vi "To Bin.vi"(8 "error in (no error)":errorcluster, 10 "s":string, 11 "n":i32) -> (0 "error out":errorcluster, 3 "Return":i32)   [LabVIEW 2010, in "TPVG_DLL.lvlib"]
doc: "This function convert an ASCII hex of 1 to four symbols to an\ninteger\n\n\nint CLASS_DECLSPEC ToBin( int, char* );"
uses:
  TPVG_DLL.lvlib
  TPVG_DLL.dll
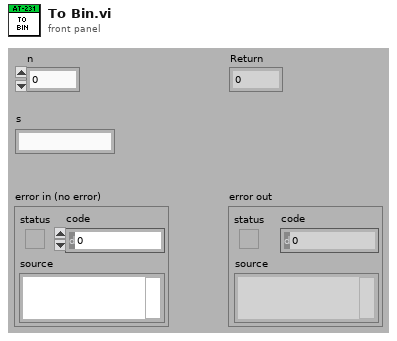
[diagram p1: front panel]
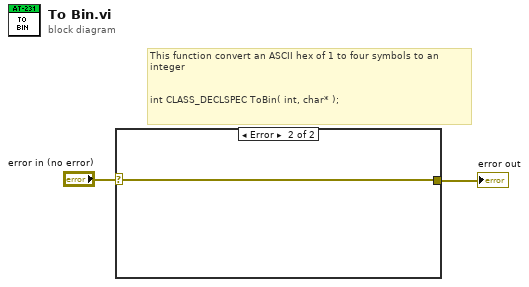
[diagram p0: block diagram]
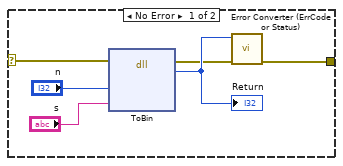
[diagram p2: hidden frame]
diagram:
  # "This function convert an ASCII hex of 1 to four symbols to an\ninteger\n\n\nint CLASS_DECLSPEC ToBin( int, char* );"
  n1 = case shown="Error" "error in (no error)" {
    selector: "error in (no error)" -> [w3 w9]
    tunnel: [w4 w9] -> w2
    frame No Error {
      n2 = dll-call lib="TPVG_DLL.*" fn="ToBin"(error in=w3, "n"="n", "s"="s") -> (error out=w5:errorcluster, "return type"=w8:i32)  [unwired: 4 in, 1 out]
      "Return" <- w8
      n3 = call "Error Converter (ErrCode or Status).vi"("error in (no error)"=w5, "error code"=w8) -> ("error out"=w4:errorcluster)  [unwired: 9 in]
    }
    frame Error {
    }
  }
  "error out" <- w2
